vi "Close Handle2.vi"(0 "handles cluster in":T1 caption="ハンドルクラスター入力", 11 "error in (no error)":errorcluster caption="エラー入力（エラーなし）") -> (4 "handles cluster out":T1 caption="ハンドルクラスター出力", 15 "error out":errorcluster caption="エラー出力")   [LabVIEW 2015]
doc: "SMTPサーバとの接続を閉じ、「Open Handle2」VIで作成したハンドルクラスターを破棄します。"
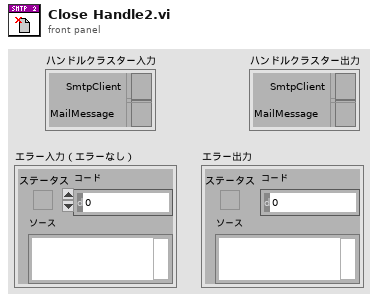
[diagram p1: front panel]
types:
  T1 = cluster{"SmtpClient":refnum<k24>, "MailMessage":refnum<k24>}
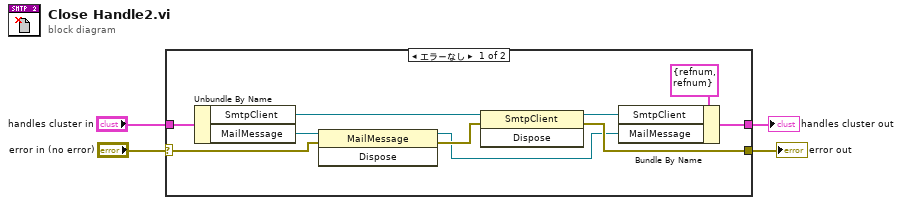
[diagram p0: block diagram]
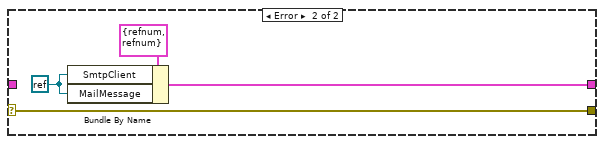
[diagram p2: hidden frame]
diagram:
  n1 = case shown="エラーなし" "error in (no error)" {
    selector: "error in (no error)" -> [w11 w18]
    tunnel: [w6 w18] -> w3
    tunnel: [w7 w15] -> w2
    tunnel: "handles cluster in" -> [w14 _]
    frame No Error {
      n2 = Unbundle By Name(w14) -> ("SmtpClient"=w13:refnum<k24>, "MailMessage"=w12:refnum<k24>)
      n3 = invoke class="MailMessage" method="Dispose"(reference=w12, error in=w11) -> (reference out=w5:refnum<k24>, error out=w10:errorcluster)  [unwired: 1 in, 1 out]
      n4 = invoke class="SmtpClient" method="Dispose"(reference=w13, error in=w10) -> (reference out=w8:refnum<k24>, error out=w6:errorcluster)  [unwired: 1 in, 1 out]
      n5 = Bundle By Name(cluster=T1 {"SmtpClient"=refnum, "MailMessage"=refnum} ("handles cluster out"), "SmtpClient"=w8, "MailMessage"=w5) -> (w7:T1)
    }
    frame Error {
      w16 = refnum<k0> refnum
      n6 = Bundle By Name(cluster=T1 {"SmtpClient"=refnum, "MailMessage"=refnum} ("handles cluster out"), "SmtpClient"=w16, "MailMessage"=w16) -> (w15:T1)
    }
  }
  "handles cluster out" <- w2
  "error out" <- w3
